vi "Step Data Buffer.vi"(6 "config paths":T1, 7 "Mode":enum16{"Init", "Read", "Write"}(ring)=enum."Write", 8 "Error In":errorcluster, 9 "Step Hisitory In":string[](array[string]), 10 "Segment Data In":T2, 11 "Add Step? In":bool) -> (0 "Error Out":errorcluster, 1 "Step Hisitory Out":string[](array[string]), 2 "Segment Data Out":T2, 3 "Add Step? Out":bool, 4 "config paths":T1)   [LabVIEW 2018]
uses:
  type defs/Sequence Info.ctl
  type defs/config paths for seq def.ctl
  type defs/Step Data Control.ctl
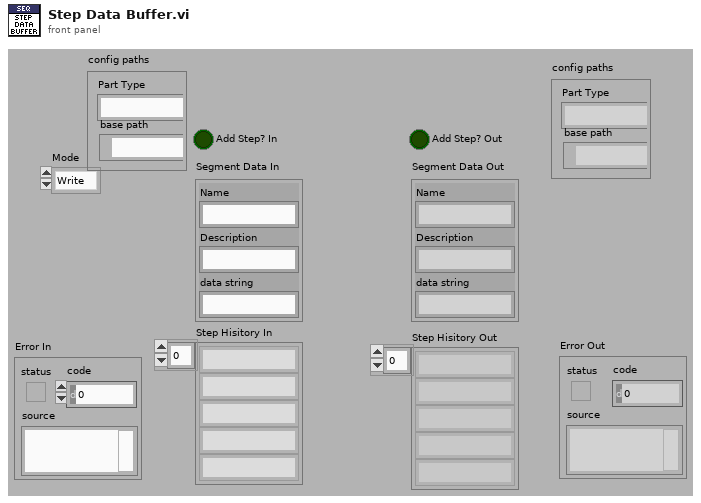
[diagram p1: front panel]
types:
  T1 = typedef "config paths for seq def.ctl" = cluster{"Part Type":string, "base path":path}
  T2 = typedef "Sequence Info.ctl" = cluster{"Name":string, "Description":string, "data string":string}
  T3 = typedef "Step Data Control.ctl" = cluster{"Add Step?":bool, "Segment Data":T2, "Step Hisitory":string[], "Part Type":string, "base path":path}
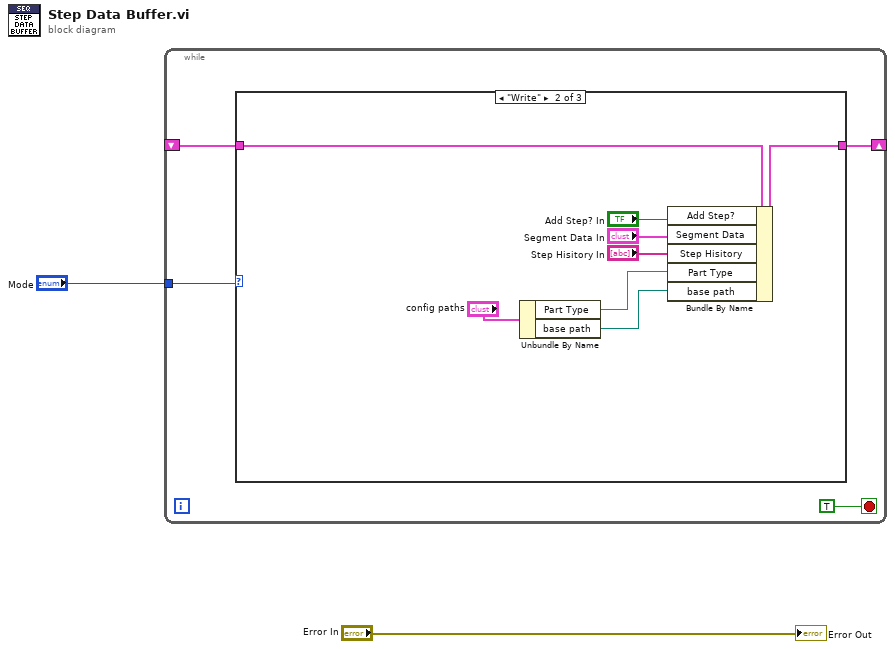
[diagram p0: block diagram]
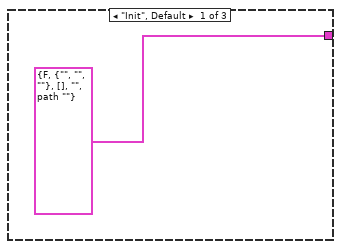
[diagram p2: hidden frame]
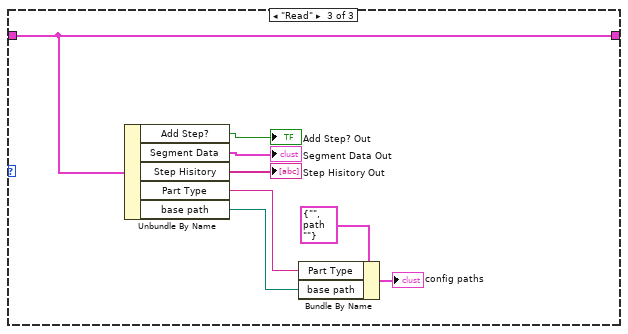
[diagram p3: hidden frame]
diagram:
  n1 = while {
    tunnel: "Mode" -> [w5]
    shift-right: [w4] -> _
    shift-left: _ -> [w3]
    stop <- TRUE stop-if-true
    n2 = case shown="\"Write\"" w5 {
      tunnel: [T3 {"Add Step?"=FALSE, "Segment Data"={"Name"="", "Description"="", "data string"=""}, "Step Hisitory"=[], "Part Type"="", "base path"=path ""} ("Step Data Control") w14 w23] -> w4
      tunnel: w3 -> [_ w15 w23]
      frame "Init", Default {
      }
      frame "Write" {
        n3 = Unbundle By Name("config paths") -> ("Part Type"=w9:string, "base path"=w8:path)
        n4 = Bundle By Name(cluster=w15, "Add Step?"="Add Step? In", "Segment Data"="Segment Data In", "Step Hisitory"="Step Hisitory In", "Part Type"=w9, "base path"=w8) -> (w14:T3)
      }
      frame "Read" {
        n5 = Unbundle By Name(w23) -> ("Add Step?"=→"Add Step? Out":bool, "Segment Data"=→"Segment Data Out":T2, "Step Hisitory"=→"Step Hisitory Out":string[], "Part Type"=w17:string, "base path"=w16:path)
        n6 = Bundle By Name(cluster=T1 {"Part Type"="", "base path"=path ""} ("config paths"), "Part Type"=w17, "base path"=w16) -> (→"config paths":T1)
      }
    }
  }
  "Error Out" <- "Error In"
